vi "OpenGraph.vi"(8 "error in (no error)":errorcluster, 11 "TAGS to show":string[](array[string])) -> (0 "Error out":errorcluster)   [LabVIEW 2020]
doc: "Open a New Gviewer graph\n\nAndre Koelewijn, 2 jan 2021\nThis vi will ask the Gserver service to open a graphic viewer.\nIf the input TAG list is used then these TAGs will show in the new graph to open.\nIf the TAG list is not wired or left empty, then a default new graph display is shown."
uses:
  Gserver/controls/Typedef_Gviewer-Query.ctl
  Gserver/controls/Typedef_QueryType.ctl
  Gserver/Gserver.lvclass
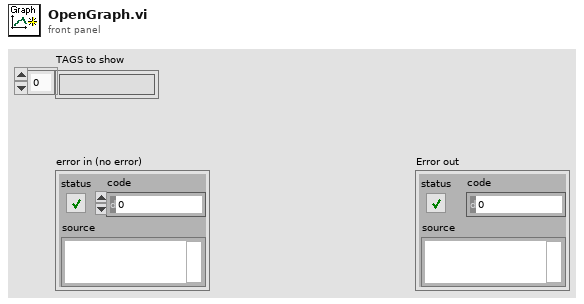
[diagram p1: front panel]
types:
  T1 = typedef "Gserver.lvclass/Typedef_QueryType.ctl" = enum16{"Subscribe", "DataRequest", "RequestAllTags", "RequestIniPath", "FAMMstarted", "SetClientOptions", "GviewerUpdate", "OpenNewGraph", "CloseClient", "CloseAllClients", "Close Gserver"}
  T2 = typedef "Gserver.lvclass/Typedef_Gviewer-Query.ctl" = cluster{"Query_type":T1, "data":variant, "Source":string, "Time Stamp":timestamp}
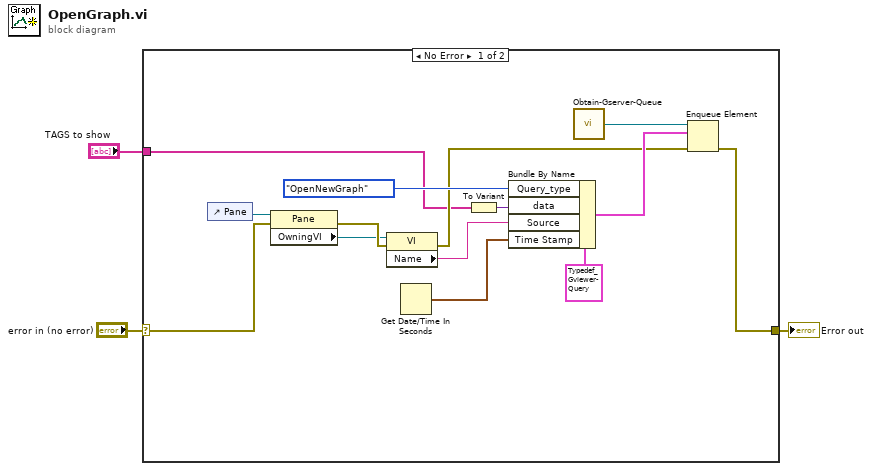
[diagram p0: block diagram]
diagram:
  n1 = case shown="No Error" "error in (no error)" {
    selector: "error in (no error)" -> [w11 w18]
    tunnel: [w8 w18] -> w2
    tunnel: "TAGS to show" -> [w6 _]
    frame No Error {
      n2 = control-ref of="Pane"() -> (w13:refnum<vi>)
      n3 = property class="Pane"(reference=w13, error in=w11) -> (error out=w10:errorcluster, "OwningVI"=w4:refnum<vi>)  [unwired: 1 out]
      n4 = property class="VI"(reference=w4, error in=w10) -> (error out=w9:errorcluster, "Name"=w12:string)  [unwired: 1 out]
      n5 = Get Date/Time In Seconds() -> (seconds since 1Jan1904=w7:timestamp)
      n6 = To Variant(anything=w6) -> (Variant=w5:variant)
      n7 = Bundle By Name(cluster=T2 {"Query_type"=enum."Subscribe", "data"=variant, "Source"="", "Time Stamp"=timestamp(0 s since 1904-01-01)} ("element"), "Query_type"=Typedef_QueryType."OpenNewGraph", "data"=w5, "Source"=w12, "Time Stamp"=w7) -> (w14:T2)
      n8 = call "Obtain-Gserver-Queue.vi"() -> ("Gserver Queue"=w17:refnum<queue>)  [unwired: 7 in]
      n9 = Enqueue Element(queue=w17, element=w14, error in (no error)=w9) -> (error out=w8:errorcluster)  [unwired: 1 in, 2 out]
    }
    frame Error {
    }
  }
  "Error out" <- w2
